vi "append_control_extimage_vihirachy.vi"() -> ()   [LabVIEW 2014]
uses:
  <vilib>/Utility/NIReport.llb/image depth.ctl
  <vilib>/Utility/NIReport.llb/Append Image to Report (path wrap).vi
  <vilib>/printing/ReportDocExtensions.llb/Append VI Hierarchy to Report (path).vi
  <vilib>/Utility/NIReport.llb/NI_report.lvclass
  <vilib>/Utility/NIReport.llb/NI_ReportGenerationCore.lvlib
panel:
  in  "VI":path
  in  "caption or alternative string":string
  in  "path or URL of image":path
  in  "image depth":T1=2 items=["B&W", "4 bits", "8 bits", "24 bits"]
  in  "template (empty)":path
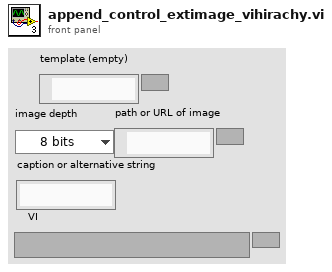
[diagram p1: front panel]
types:
  T1 = typedef "NI_ReportGenerationCore.lvlib/image depth.ctl" = u16
  T2 = enum16{"Standard Report", "HTML", "Word", "Excel"}
  T3 = enum16{"maximized", "minimized", "normal", "no change"}
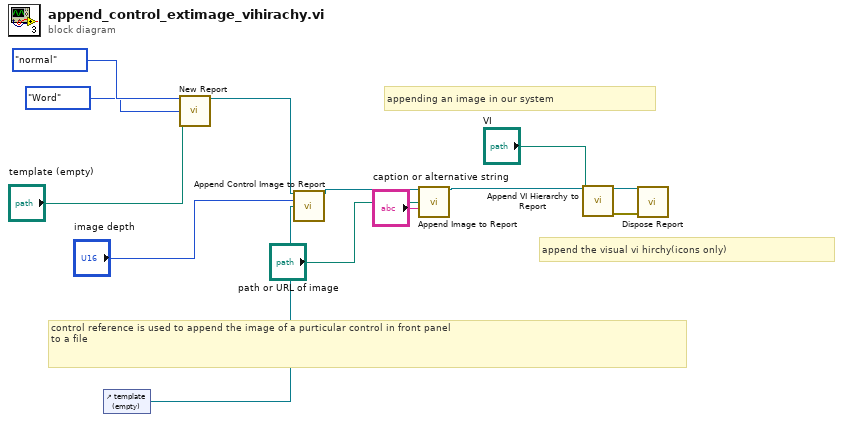
[diagram p0: block diagram]
diagram:
  # "append the visual vi hirchy(icons only)"
  # "appending an image in our system"
  # "control reference is used to append the image of a purticular control in front panel\nto a file"
  n1 = control-ref of="template (empty)"() -> (w3:refnum<vi>)
  n2 = call <vilib>:"New Report.vi"("window state (normal)"=T3."normal", "report type"=T2."Word", "template (empty)"="template (empty)") -> ("report out"=w8:refnum<class "NI_report.lvclass">)  [unwired: 11 in, 1 out]
  n3 = call-dynamic "Append Control Image to Report.vi"("report in"=w8, "image depth"="image depth", "ctrl reference"=w3) -> ("report out"=w12:refnum<class "NI_report.lvclass">)  [unwired: 9 in, 3 out]
  n4 = call-poly <vilib>:"Append Image to Report.vi"("report in"=w12, "path or URL of image"="path or URL of image", "caption or alternative string"="caption or alternative string") -> ("report out"=w13:refnum<class "NI_report.lvclass">)  [unwired: 9 in, 3 out]
  n5 = call-poly <vilib>:"Append VI Hierarchy to Report.vi"("report in"=w13, "VI"="VI") -> ("report out"=w2:refnum<class "NI_report.lvclass">, "error out"=w1:errorcluster)  [unwired: 9 in, 3 out]
  n6 = call-dynamic "Dispose Report.vi"("report in"=w2, "error in (no error)"=w1) -> ()  [unwired: 13 in, 1 out]
